vi "DieMatch.vi"() -> ()   [LabVIEW 2015]
panel:
  out "# of Rolls":dbl
  out "Die 2":dbl
  out "Die 1":dbl
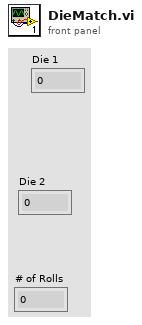
[diagram p1: front panel]
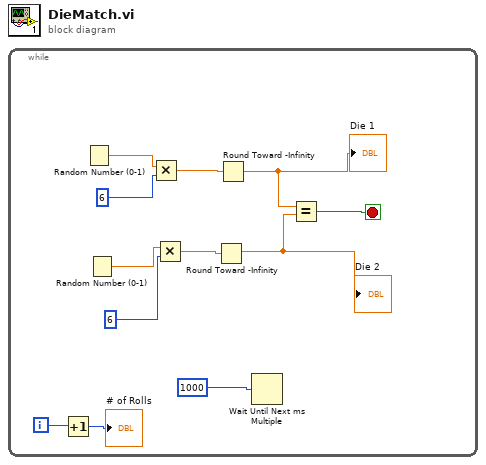
[diagram p0: block diagram]
diagram:
  n1 = while {
    i -> [w11]
    stop <- w1 stop-if-true
    n2 = Increment(x=w11) -> (x+1=→"# of Rolls":i32)
    n3 = Random Number (0-1)() -> (number: 0 to 1=w9:dbl)
    n4 = Random Number (0-1)() -> (number: 0 to 1=w5:dbl)
    n5 = Multiply(x=w9, y=6) -> (x*y=w7:dbl)
    n6 = Multiply(x=w5, y=6) -> (x*y=w3:dbl)
    n7 = Round Toward -Infinity(1:w3) -> (0:w2:dbl)
    "Die 2" <- w2
    n8 = Round Toward -Infinity(1:w7) -> (0:w6:dbl)
    "Die 1" <- w6
    n9 = Wait Until Next ms Multiple(millisecond multiple=1000) -> ()  [unwired: 1 out]
    n10 = Equal?(x=w6, y=w2) -> (x = y?=w1:bool)
  }
